vi "AE Camera April Tag Image.vi"(7 "Update":bool, 11 "Ball Image in":T1(plugin-control)=refnum) -> (3 "Ball Image out":T1(plugin-control))   [LabVIEW 2023]
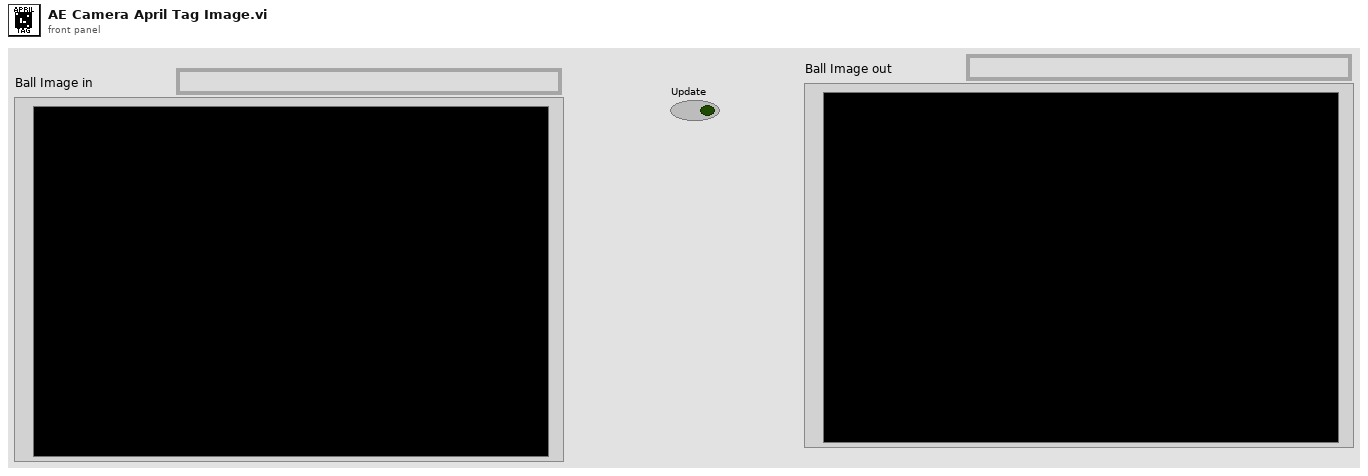
[diagram p1: front panel]
types:
  T1 = typedef "IMAQ Image.ctl" = refnum<image>
  T2 = typedef "Image Type" = u32
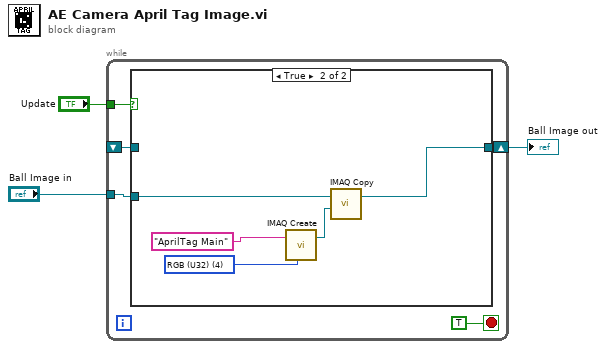
[diagram p0: block diagram]
diagram:
  n1 = while {
    tunnel: "Update" -> [w8]
    tunnel: "Ball Image in" -> [w7]
    shift-right: [w6] -> w1
    shift-left: _ -> [w5]
    stop <- TRUE stop-if-true
    n2 = case shown="True" w8 {
      tunnel: w7 -> [_ w14]
      tunnel: [w9 w13] -> w6
      tunnel: w5 -> [w9 _]
      frame False {
      }
      frame True {
        w12 = T2 4 items=["Grayscale (U8)", "Grayscale (I16)", "Grayscale (SGL)", "Complex (CSG)", "RGB (U32)", "HSL (U32)", "RGB (U64)", "Grayscale (U16)"] ("Image Type")
        n3 = call "IMAQ Create"("Image Name"="AprilTag Main" ("string"), "Image Type"=w12) -> ("New Image"=w11:T1)  [unwired: 2 in, 2 out]
        n4 = call "IMAQ Copy"("Image Dst"=w11, "Image Src"=w14) -> ("Image Dst Out"=w13:T1)  [unwired: 4 in, 1 out]
      }
    }
  }
  "Ball Image out" <- w1
